vi "Orb_Register.vi"(0 "error in (no error)":errorcluster, 6 "Registering VI":string) -> (3 "error out":errorcluster)   [LabVIEW 2009]
uses:
  Orb_Global.vi
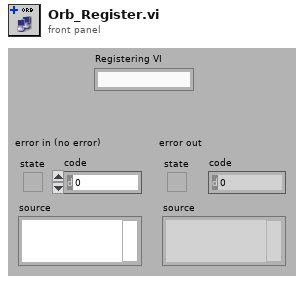
[diagram p1: front panel]
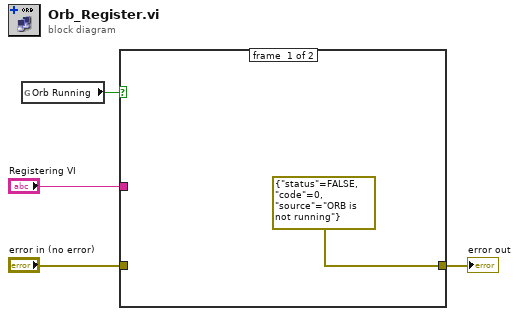
[diagram p0: block diagram]
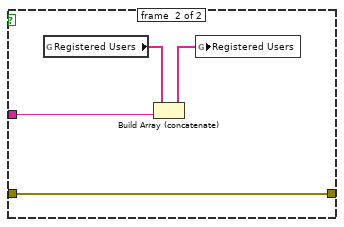
[diagram p2: hidden frame]
diagram:
  n1 = global read "Orb_Global.vi" "Orb Running"() -> (w3:bool)
  n2 = case shown="True" w3 {
    tunnel: "error in (no error)" -> [_ w9]
    tunnel: [errorcluster {"status"=FALSE, "code"=0, "source"="ORB is not running"} ("error out") w9] -> w2
    tunnel: "Registering VI" -> [_ w8]
    frame #0 {
    }
    frame #1 {
      n3 = global read "Orb_Global.vi" "Registered Users"() -> (w7:string[])
      n4 = Build Array (concatenate)(w7, w8) -> (w6:string[])
      n5 = global write "Orb_Global.vi" "Registered Users"(w6) -> ()
    }
  }
  "error out" <- w2
